vi "I2C Write.vi"(7 "I2C Channel (0)":u8, 8 "Error In":errorcluster, 9 "Data":u8[](array[numeric]), 10 "I2C Slave Address":u8, 11 "LINX Device Config":T1) -> (0 "Error Out":errorcluster, 3 "LINX Device Config":T1)   [LabVIEW 2011, in "LVH-LINX.lvlib" / "Device.lvlib"]
doc: "Write one or more bytes on the specified I2C channel."
uses:
  Device.lvlib
  Type Defs/LINX Device Config.ctl
  Type Defs/Interface.ctl
  Type Defs/TCP Config.ctl
  Type Defs/Device Family.ctl
  Type Defs/Error Type.ctl
  LVH-LINX.lvlib
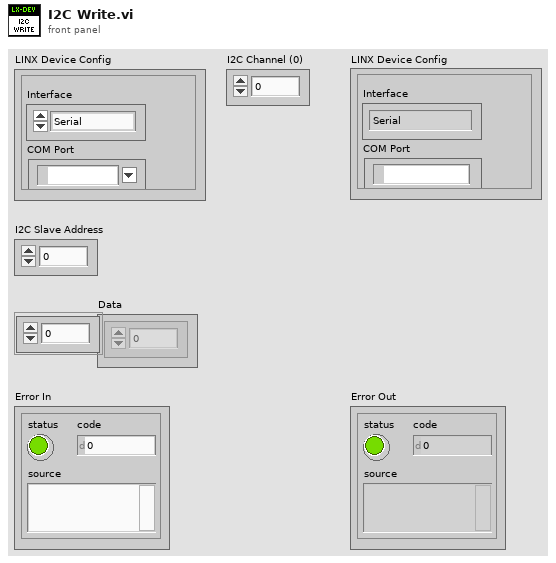
[diagram p1: front panel]
types:
  T1 = typedef "LVH-LINX.lvlib/Device.lvlib/LINX Device Config.ctl" = cluster{"Interface":T2, "COM Port":refnum<visa-resource-name>, "TCP Configuration":T3, "Device Family":T4, "Device ID":u8, "Device Name":string, "TCP Ref":refnum<k5>}
  T2 = typedef "LVH-LINX.lvlib/Interface.ctl" = enum16{"Serial", "TCP"}
  T3 = typedef "LVH-LINX.lvlib/Device.lvlib/TCP Config.ctl" = cluster{"IP Address":string, "Port":u16}
  T4 = typedef "LVH-LINX.lvlib/Device Family.ctl" = enum8{"National Instruments", "Digilent", "Arduino"}
  T5 = typedef "LVH-LINX.lvlib/Error Type.ctl" = enum16{"Unknown", "Timeout", "Corrupt Return Packet", "Unable To Connect", "Command Not Supported", "Channel DNE"}
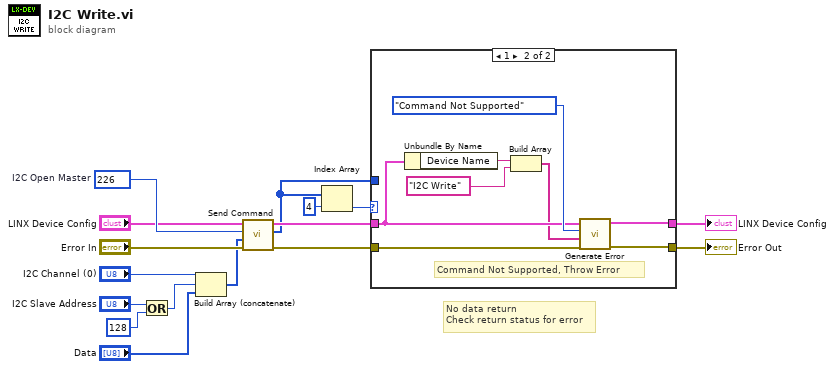
[diagram p0: block diagram]
diagram:
  w15 = u16 226  # I2C Open Master
  # "No data return\nCheck return status for error"
  n1 = Or(x="I2C Slave Address", y=u8 128) -> (x .or. y?=w2:u8)
  n2 = Build Array (concatenate)("I2C Channel (0)", w2, "Data") -> (w6:u8[])
  n3 = call "Send Command.vi"("Error In"="Error In", "ARGS"=w6, "CMD"=w15, "LINX Device Config"="LINX Device Config") -> ("Error Out"=w8:errorcluster, "Response"=w7:u8[], "LINX Device Config"=w10:T1)  [unwired: 5 in]
  n4 = Index Array(array=w7, index=4) -> (element=w12:u8)
  n5 = case shown="1" w12 {
    tunnel: [w18 w24] -> w11
    tunnel: w10 -> [w18 w22]
    tunnel: [w17 w25] -> w9
    tunnel: w8 -> [w17 w26]
    tunnel: w7 -> [_ _]
    frame 0, Default {
      # "Status OK, Process Data"
    }
    frame 1 {
      # "Command Not Supported, Throw Error"
      n6 = Unbundle By Name(w22) -> ("Device Name"=w21:string)
      n7 = Build Array(w21, "I2C Write") -> (w19:string[])
      n8 = call "Generate Error.vi"("Error In"=w26, "Arguments"=w19, "Error Type"=Error_Type."Command Not Supported", "LINX Device Config"=w22) -> ("Error Out"=w25:errorcluster, "LINX Device Config"=w24:T1)  [unwired: 6 in]
    }
  }
  "Error Out" <- w9
  "LINX Device Config" <- w11
